vi "Build Tree.vi"(6 "Show IDs":bool, 7 "Linked List ID":string, 8 "error in (no error)":errorcluster, 9 "Tag Blacklist":i8[](array[numeric]), 11 "Linked List Ref":refnum<data-value>) -> (0 "error out":errorcluster, 2 "Tree Data":T1(array[cluster]), 3 "Linked List Ref out":refnum<data-value>)   [LabVIEW 2019, in "Linked Lists.lvlib" / "Linked List Ref.lvclass"]
uses:
  <vilib>/gpm_packages/@cs/linked-list/Source/Linked List/Linked List Ref/Linked List Ref.lvclass
  <vilib>/gpm_packages/@cs/linked-list/Source/Linked List/ILinkedList/ILinked List.lvclass
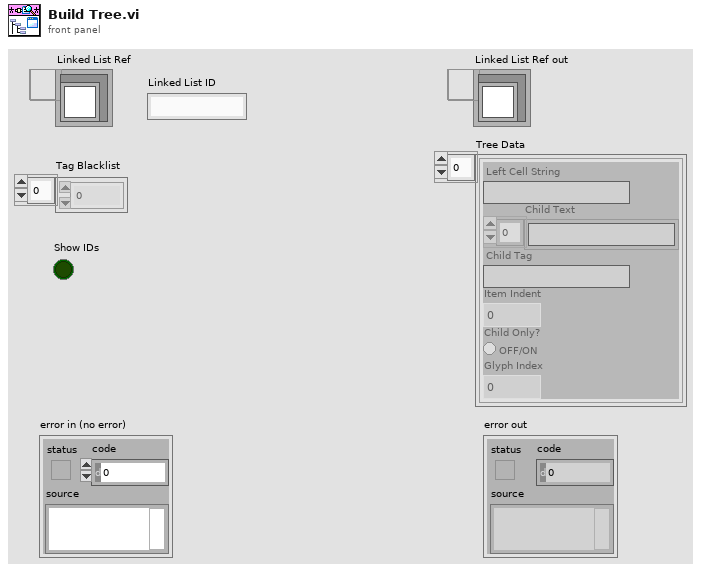
[diagram p1: front panel]
types:
  T1 = cluster{"Left Cell String":string, "Child Text":string[], "Child Tag":string, "Item Indent":i32, "Child Only?":bool, "Glyph Index":i32}[]
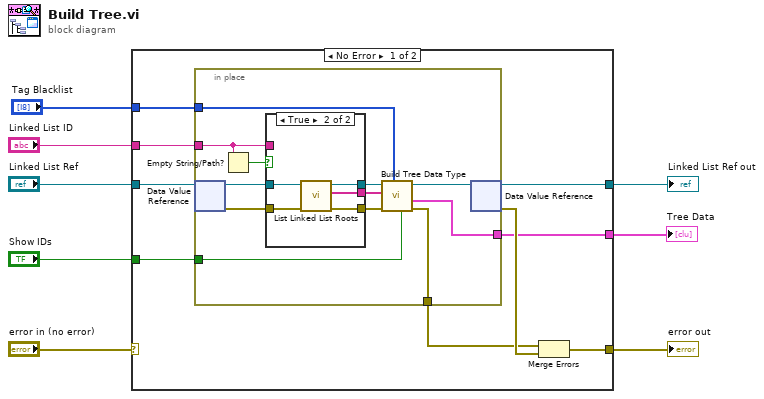
[diagram p0: block diagram]
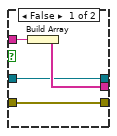
[diagram p2: hidden frame]
diagram:
  n1 = case shown="No Error" "error in (no error)" {
    selector: "error in (no error)" -> [_ w40]
    tunnel: "Linked List Ref" -> [w17 w39]
    tunnel: "Linked List ID" -> [w16 _]
    tunnel: [w14 w40] -> w5
    tunnel: [w15 w39] -> w4
    tunnel: "Show IDs" -> [w11 _]
    tunnel: [w10 _] -> w2
    tunnel: "Tag Blacklist" -> [w9 _]
    frame No Error {
      n2 = in-place {
        in-place-border: w16 -> [w23]
        in-place-border: [w28] -> w12
        in-place-border: w11 -> [w26]
        in-place-border: [w25] -> w10
        in-place-border: w9 -> [w24]
        n3 = in-place-dvr #1(w17) -> (w21:refnum<class "ILinked List.lvclass">, w19:errorcluster)
        n4 = Empty String/Path?(string/path=w23) -> (empty?=w22:bool)
        n5 = case shown="True" w22 {
          tunnel: [w33 w34] -> w27
          tunnel: w23 -> [w32 _]
          tunnel: [w31 w35] -> w20
          tunnel: w21 -> [w31 w36]
          tunnel: [w30 w37] -> w18
          tunnel: w19 -> [w30 w38]
          frame False {
            n6 = Build Array(w32) -> (w33:string[])
          }
          frame True {
            n7 = call-dynamic "List Linked List Roots.vi"("error in (no error)"=w38, "ILinked List in"=w36) -> ("error out"=w37:errorcluster, "Root IDs"=w34:string[], "ILinked List out"=w35:refnum<class "ILinked List.lvclass">)  [unwired: 6 in, 1 out]
          }
        }
        n8 = call-dynamic "Build Tree Data Type.vi"("Show IDs (True)"=w26, "Tag Blacklist"=w24, "error in (no error)"=w18, "Child IDs"=w27, "ILinked List in"=w20) -> ("error out"=w28:errorcluster, "Items Out"=w25:T1, "ILinked List out"=w29:refnum<class "ILinked List.lvclass">)  [unwired: 4 in]
        n9 = in-place-dvr #1(w29) -> (w15:refnum<data-value>, w13:errorcluster)
      }
      n10 = Merge Errors(w12, w13) -> (w14:errorcluster)
    }
    frame Error {
    }
  }
  "error out" <- w5
  "Linked List Ref out" <- w4
  "Tree Data" <- w2
